vi "Batch rename files.vi"() -> ()   [LabVIEW 2020]
panel:
  out "length":i32
  out "Files renamed":i32
  out "Files found":i32
  in  "Numeric Control":i32=5
  in  "File extension (empty=don't care)":string
  in  "save":bool
  in  "file name must include":string
  in  "File Path Control":path=path "\\\\wispryinc.net\\dfs/Home/Niko.Kuusniemi/My Documents/WS5100 SP4T/Measurements/180920 HB Harmonics"
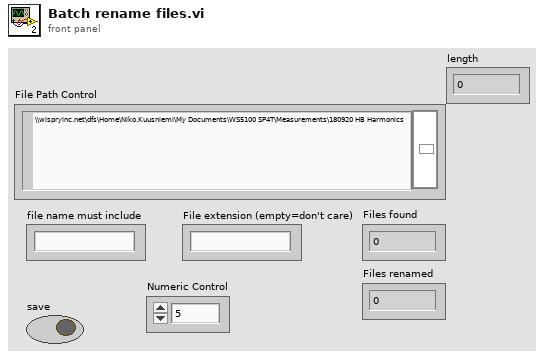
[diagram p1: front panel]
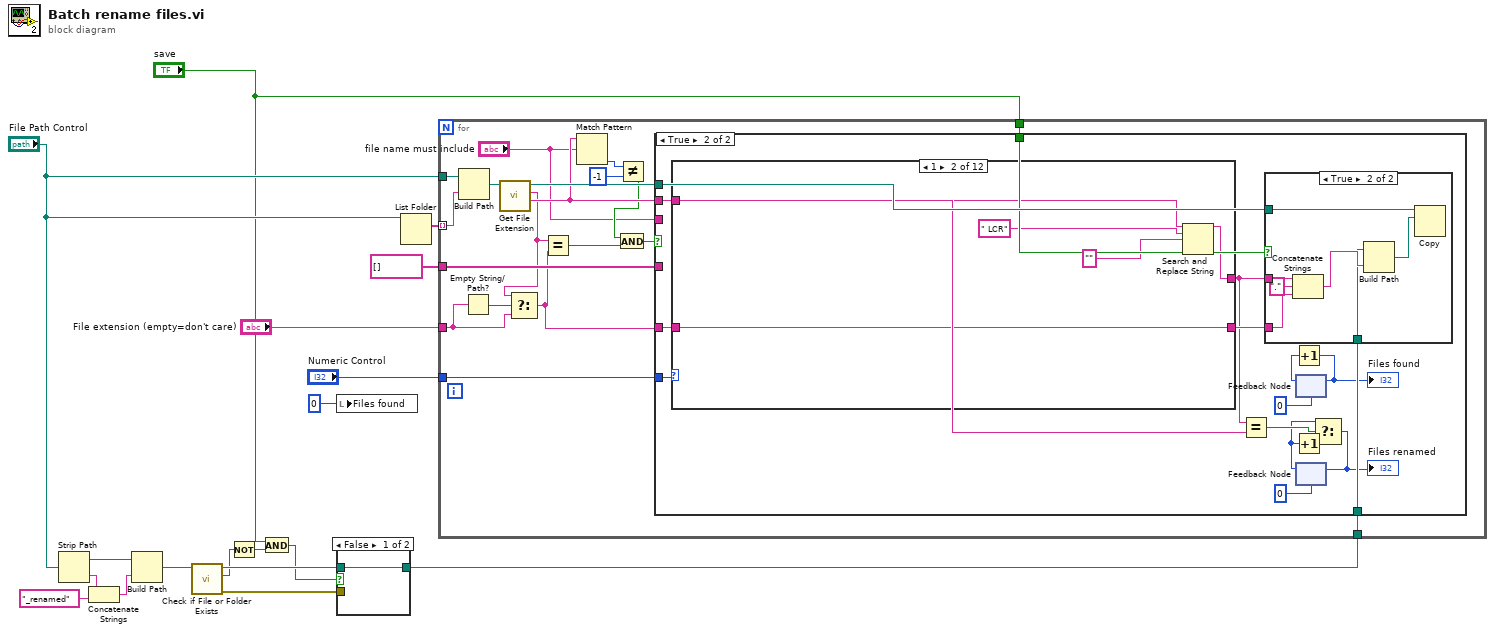
[diagram p0: block diagram]
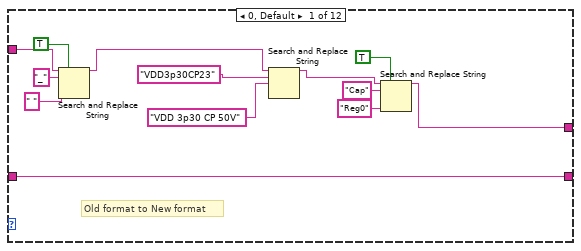
[diagram p3: hidden frame]
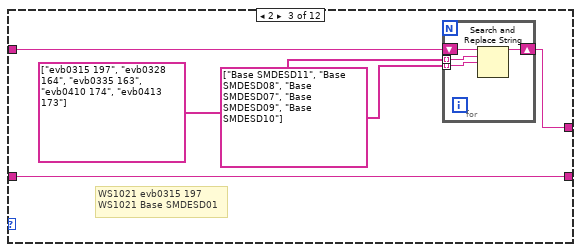
[diagram p4: hidden frame]
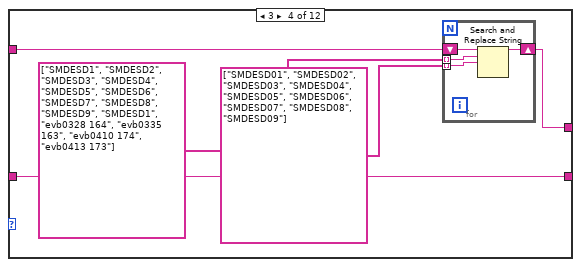
[diagram p5: hidden frame]
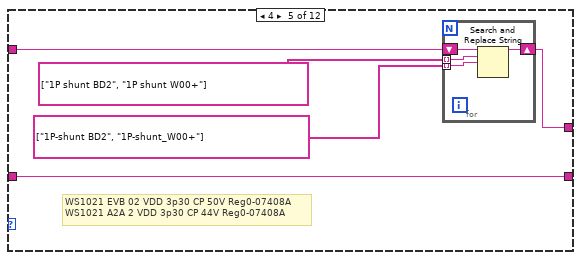
[diagram p6: hidden frame]
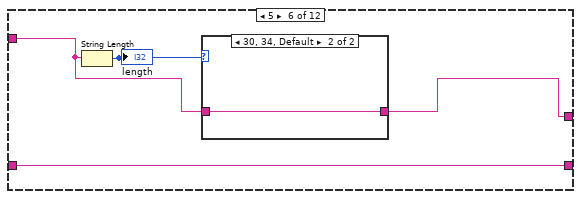
[diagram p7: hidden frame]
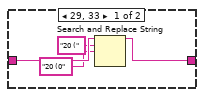
[diagram p8: hidden frame]
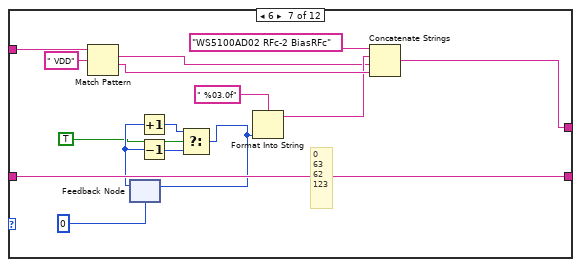
[diagram p9: hidden frame]
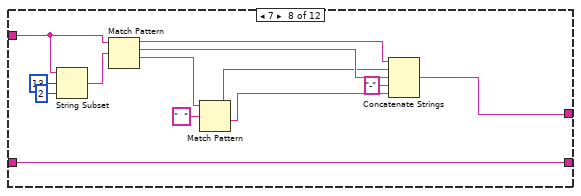
[diagram p10: hidden frame]
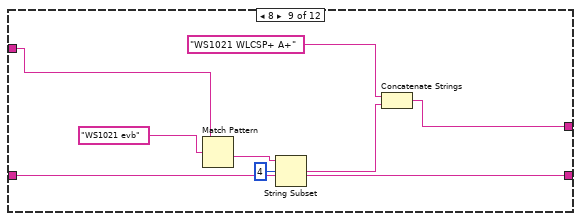
[diagram p11: hidden frame]
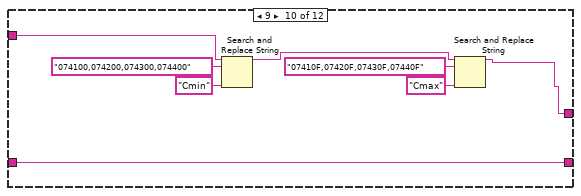
[diagram p12: hidden frame]
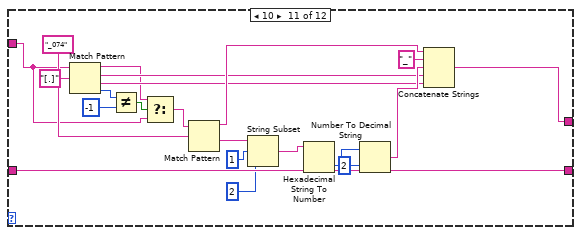
[diagram p13: hidden frame]
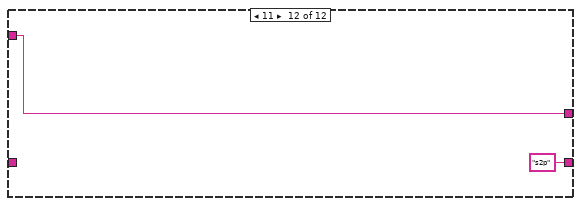
[diagram p14: hidden frame]
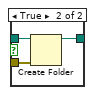
[diagram p16: hidden frame]
diagram:
  n1 = Strip Path(path="File Path Control") -> (stripped path=w14:path, name=w17:string)
  n2 = Concatenate Strings(w17, "_renamed" ("string")) -> (w15:string)
  n3 = Build Path(base path=w14, name or relative path=w15) -> (appended path=w13:path)
  n4 = call <vilib>:"Check if File or Folder Exists.vi"("path"=w13) -> ("error out"=w11:errorcluster, "file or folder exists?"=w6:bool, "dup path"=w12:path)  [unwired: 8 in]
  n5 = Not(x=w6) -> (.not. x?=w5:bool)
  n6 = And(x="save", y=w5) -> (x .and. y?=w7:bool)
  n7 = local write "Files found"(0 ("Files renamed")) -> ()
  n8 = case shown="False" w7 {
    tunnel: [w19 w22] -> w8
    tunnel: w12 -> [w19 w21]
    tunnel: w11 -> [_ w20]
    frame False {
    }
    frame True {
      n9 = Create Folder(path (use dialog)=w21, error in=w20) -> (created path=w22:path)  [unwired: 1 in, 2 out]
    }
  }
  n10 = List Folder(path="File Path Control") -> (filenames=w10:string[])  [unwired: 3 in, 3 out]
  n11 = for {
    tunnel: "File Path Control" -> [w41]
    tunnel: w10 -> [w37] mode=indexing
    tunnel: string[] [] -> [w40]
    tunnel: w8 -> [w36]
    tunnel: "save" -> [w28]
    tunnel: "File extension (empty=don't care)" -> [w25]
    tunnel: "Numeric Control" -> [w27]
    n12 = Build Path(base path=w41, name or relative path=w37) -> (appended path=w39:path)
    n13 = Empty String/Path?(string/path=w25) -> (empty?=w26:bool)
    n14 = call <vilib>:"Get File Extension.vi"("file"=w39) -> ("filename without extension"=w33:string, "lowercase file extension"=w23:string, "dup file"=w38:path)  [unwired: 6 in, 2 out]
    n15 = Select(t=w23, s=w26, f=w25) -> (s? t:f=w24:string)
    n16 = Equal?(x=w23, y=w24) -> (x = y?=w35:bool)
    n17 = Match Pattern(string=w33, regular expression="file name must include") -> (offset past match=w32:i32)  [unwired: 1 in, 3 out]
    n18 = Not Equal?(x=w32, y=-1) -> (x != y?=w30:bool)
    n19 = And(x=w30, y=w35) -> (x .and. y?=w34:bool)
    n20 = case shown="True" w34 {
      tunnel: w33 -> [_ w48]
      tunnel: w40 -> [_ _]
      tunnel: w38 -> [_ w57]
      tunnel: w36 -> [_ w56]
      tunnel: w24 -> [_ w53]
      tunnel: "file name must include" -> [_ _]
      tunnel: w28 -> [_ w55]
      tunnel: w27 -> [_ w54]
      frame False {
      }
      frame True {
        n21 = case shown="1" w54 {
          tunnel: w48 -> [w66 w75 w80 w89 w98 w104 w124 w136 w142 w155 w156 w178]
          tunnel: [w62 w74 w79 w88 w97 w103 w125 w127 w140 w148 w162 w178] -> w49
          tunnel: w53 -> [w58 w73 w78 w87 w96 w106 w126 w139 w147 w154 w176 _]
          tunnel: [w58 w73 w78 w87 w96 w106 w126 w139 w147 w154 w176 "s2p" ("File extension (empty=don't care)")] -> w52
          frame 0, Default {
            # "Old format to New format"
            n22 = Search and Replace String(replace all?=TRUE ("replace all? (F)"), input string=w66, search string="_", replace string=" " ("replace string (\"\")")) -> (result string=w65:string)  [unwired: 4 in, 3 out]
            n23 = Search and Replace String(input string=w65, search string="VDD3p30CP23", replace string="VDD 3p30 CP 50V" ("replace string (\"\")")) -> (result string=w63:string)  [unwired: 5 in, 3 out]
            n24 = Search and Replace String(replace all?=TRUE ("replace all? (F)"), input string=w63, search string="Cap", replace string="Reg0" ("replace string (\"\")")) -> (result string=w62:string)  [unwired: 4 in, 3 out]
          }
          frame 1 {
            n25 = Search and Replace String(input string=w75, search string=" LCR", replace string="" ("search string")) -> (result string=w74:string)  [unwired: 5 in, 3 out]
          }
          frame 2 {
            # "WS1021 evb0315 197\nWS1021 Base SMDESD01"
            n26 = for {
              tunnel: string[] ["Base SMDESD11", "Base SMDESD08", "Base SMDESD07", "Base SMDESD09", "Base SMDESD10"] -> [w82] mode=indexing
              tunnel: string[] ["evb0315 197", "evb0328 164", "evb0335 163", "evb0410 174", "evb0413 173"] -> [w81] mode=indexing
              shift-right: [w83] -> w79
              shift-left: w80 -> [w84]
              n27 = Search and Replace String(input string=w84, search string=w81, replace string=w82) -> (result string=w83:string)  [unwired: 5 in, 3 out]
            }
          }
          frame 3 {
            n28 = for {
              tunnel: string[] ["SMDESD01", "SMDESD02", "SMDESD03", "SMDESD04", "SMDESD05", "SMDESD06", "SMDESD07", "SMDESD08", "SMDESD09"] -> [w91] mode=indexing
              tunnel: string[] ["SMDESD1", "SMDESD2", "SMDESD3", "SMDESD4", "SMDESD5", "SMDESD6", "SMDESD7", "SMDESD8", "SMDESD9", "SMDESD1", "evb0328 164", "evb0335 163", "evb0410 174", "evb0413 173"] -> [w90] mode=indexing
              shift-right: [w92] -> w88
              shift-left: w89 -> [w93]
              n29 = Search and Replace String(input string=w93, search string=w90, replace string=w91) -> (result string=w92:string)  [unwired: 5 in, 3 out]
            }
          }
          frame 4 {
            # "WS1021 EVB 02 VDD 3p30 CP 50V Reg0-07408A\nWS1021 A2A 2 VDD 3p30 CP 44V Reg0-07408A"
            n30 = for {
              tunnel: string[] ["1P-shunt BD2", "1P-shunt_W00+"] -> [w100] mode=indexing
              tunnel: string[] ["1P shunt BD2", "1P shunt W00+"] -> [w99] mode=indexing
              shift-right: [w101] -> w97
              shift-left: w98 -> [w102]
              n31 = Search and Replace String(input string=w102, search string=w99, replace string=w100) -> (result string=w101:string)  [unwired: 5 in, 3 out]
            }
          }
          frame 5 {
            n32 = String Length(string=w104) -> (length=w105:i32)
            "length" <- w105
            n33 = case shown="30, 34, Default" w105 {
              tunnel: [w107 w111] -> w103
              tunnel: w104 -> [w110 w111]
              frame 29, 33 {
                n34 = Search and Replace String(input string=w110, search string="20 (", replace string="20 (0" ("search string")) -> (result string=w107:string)  [unwired: 5 in, 3 out]
              }
              frame 30, 34, Default {
              }
            }
          }
          frame 6 {
            # "0\n63\n62\n123"
            n35 = Match Pattern(string=w124, regular expression=" VDD") -> (match substring=w117:string, after substring=w122:string)  [unwired: 1 in, 2 out]
            n36 = feedback #1(0) -> (w116:i32)
            n37 = Increment(x=w116) -> (x+1=w113:i32)
            n38 = Decrement(x=w116) -> (x-1=w115:i32)
            n39 = Select(t=w113, s=TRUE, f=w115) -> (s? t:f=w112:i32)
            n40 = feedback-in #1(w112) -> ()
            n41 = Format Into String(format string=" %03.0f", w112) -> (resulting string=w118:string)  [unwired: 2 in, 1 out]
            n42 = Concatenate Strings("WS5100AD02 RFc-2 BiasRFc" ("string"), w118, w117, w122) -> (w125:string)
          }
          frame 7 {
            n43 = String Subset(string=w136, offset (0)=13, length (rest)=2 ("length (rest)")) -> (substring=w137:string)
            n44 = Match Pattern(string=w136, regular expression=w137) -> (before substring=w135:string, match substring=w130:string, after substring=w132:string)  [unwired: 1 in, 1 out]
            n45 = Match Pattern(string=w132, regular expression="  ") -> (before substring=w129:string, after substring=w131:string)  [unwired: 1 in, 2 out]
            n46 = Concatenate Strings(w135, w129, w130, "-" ("string"), w131) -> (w127:string)
          }
          frame 8 {
            n47 = Match Pattern(string=w142, regular expression="WS1021 evb" ("search string")) -> (after substring=w146:string)  [unwired: 1 in, 3 out]
            n48 = String Subset(string=w146, offset (0)=4) -> (substring=w141:string)  [unwired: 1 in]
            n49 = Concatenate Strings("WS1021 WLCSP+ A+" ("replace string (\"\")"), w141) -> (w140:string)
          }
          frame 9 {
            n50 = Search and Replace String(input string=w155, search string="074100,074200,074300,074400", replace string="Cmin" ("replace string (\"\")")) -> (result string=w149:string)  [unwired: 5 in, 3 out]
            n51 = Search and Replace String(input string=w149, search string="07410F,07420F,07430F,07440F", replace string="Cmax" ("replace string (\"\")")) -> (result string=w148:string)  [unwired: 5 in, 3 out]
          }
          frame 10 {
            n52 = Match Pattern(string=w156, regular expression="[.]") -> (before substring=w158:string, match substring=w164:string, after substring=w163:string, offset past match=w161:i32)  [unwired: 1 in]
            n53 = Not Equal?(x=w161, y=-1) -> (x != y?=w159:bool)
            n54 = Select(t=w158, s=w159, f=w156) -> (s? t:f=w157:string)
            n55 = Match Pattern(string=w157, regular expression="_074") -> (before substring=w169:string, after substring=w174:string)  [unwired: 1 in, 2 out]
            n56 = String Subset(string=w174, offset (0)=1, length (rest)=2 ("offset (0)")) -> (substring=w171:string)
            n57 = Hexadecimal String To Number(string=w171) -> (number=w170:u32)  [unwired: 2 in, 1 out]
            n58 = Number To Decimal String(number=w170, width (-)=i16 2) -> (decimal integer string=w165:string)
            n59 = Concatenate Strings(w169, "_" ("string"), w165, w164, w163) -> (w162:string)
          }
          frame 11 {
          }
        }
        n60 = Equal?(x=w49, y=w48) -> (x = y?=w45:bool)
        n61 = case shown="True" w55 {
          tunnel: w57 -> [_ w185]
          tunnel: w49 -> [_ w184]
          tunnel: w56 -> [_ w182]
          tunnel: w52 -> [_ w180]
          frame False {
          }
          frame True {
            n62 = Concatenate Strings(w184, "." ("string"), w180) -> (w183:string)
            n63 = Build Path(base path=w182, name or relative path=w183) -> (appended path=w181:path)
            n64 = Copy(10:w181, 11:w185) -> ()  [unwired: 3 in, 3 out]
          }
        }
        n65 = feedback #2(0) -> (w51:i32)
        n66 = Increment(x=w51) -> (x+1=w50:i32)
        "Files found" <- w50
        n67 = feedback-in #2(w50) -> ()
        n68 = feedback #3(0) -> (w43:i32)
        n69 = Increment(x=w43) -> (x+1=w44:i32)
        n70 = Select(t=w43, s=w45, f=w44) -> (s? t:f=w42:i32)
        "Files renamed" <- w42
        n71 = feedback-in #3(w42) -> ()
      }
    }
  }
